vi "Close Connection.vi"(8 "error in (no error)":errorcluster, 11 "NI-9421 (C Series) in":refnum<class "NI-9421 (C Series).lvclass">) -> (0 "error out":errorcluster, 3 "NI-9421 (C Series) out":refnum<class "NI-9421 (C Series).lvclass">)   [LabVIEW 2020, in "NI-9421 (C Series).lvclass"]
uses:
  NI-9421 (C Series).lvclass
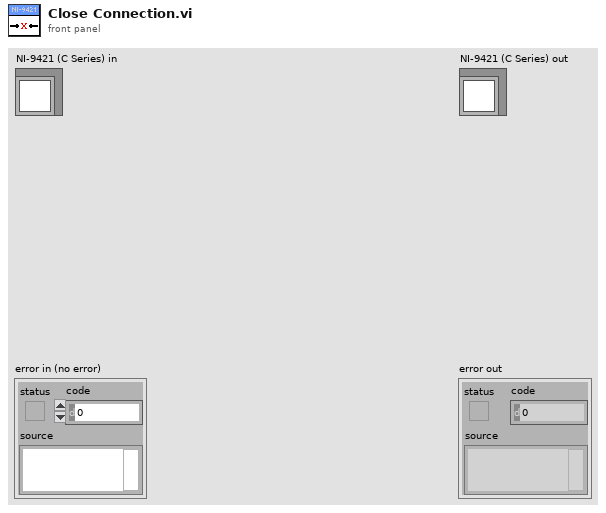
[diagram p1: front panel]
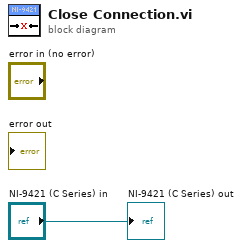
[diagram p0: block diagram]
diagram:
  "NI-9421 (C Series) out" <- "NI-9421 (C Series) in"
